vi "Client Init Test.vi"() -> (0 "no error":errorcluster, 1 "tags found":bool, 2 "expected execution settings":bool)   [LabVIEW 2013, in "OPC UA Client Tests.lvlib"]
doc: "Tests Init override for server configuration"
uses:
  OPC UA Client Tests.lvlib
  <vilib>/NI/Tag Bus/dictionary/data dictionary.lvclass
  module/configuration/OPC UA Client configuration.lvclass
  <vilib>/opcua/NI OPC UA Server.lvlib
  module/execution/OPC UA Client runtime.lvclass
  <vilib>/OPCUA/server/subVI/supported security policies.ctl
  <vilib>/NI/Tag Bus Module Framework/channel/TBM channel.lvclass
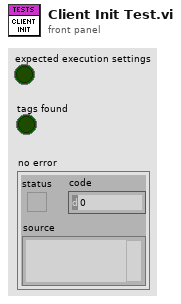
[diagram p1: front panel]
types:
  T1 = typedef "supported security policies.ctl" = cluster{"None":bool, "Sign with Basic128Rsa125":bool, "Sign and Encrypt with Basic128Rsa125":bool, "Sign with Basic256":bool, "Sign and Encrypt with Basic256":bool}
  T2 = cluster{"Client?":bool, "Server Certificates":cluster{"Relative Path?":bool, "Certificate Paths":path[], "Certificate Names":string[]}, "Client Certificates":cluster{"Relative Path?":bool, "Certificate Paths":path[], "Certificate Names":string[]}, "Client Configuration":cluster{"Server Endpoint URL":string, "Security Policy":cluster{"Message Mode":enum16{"None", "Sign", "Sign and Encrypt"}, "Security":enum16{"Basic256", "Basic128Rsa15"}}, "Username/Password":cluster{"Username":string, "Password":string}}, "Server Configuration":cluster{"Server Name":string, "TCP port (49580)":string, "Supported Security Policies":T1}}
  T3 = cluster{"Server Certificates":cluster{"Relative Path?":bool, "Certificate Paths":path[], "Certificate Names":string[]}, "Client Certificates":cluster{"Relative Path?":bool, "Certificate Paths":path[], "Certificate Names":string[]}, "Client Configuration":cluster{"Server Endpoint URL":string, "Security Policy":cluster{"Message Mode":enum16{"None", "Sign", "Sign and Encrypt"}, "Security":enum16{"Basic256", "Basic128Rsa15"}}, "Username/Password":cluster{"Username":string, "Password":string}}}
  T4 = typedef "OPC UA configuration.lvclass/Line.ctl" = cluster{"channel":refnum<class "TBM channel.lvclass">, "Node Path":string, "OPC UA Data Type":T5}
  T5 = typedef "OPC UA configuration.lvclass/OPC UA Data Type.ctl" = u16
  T6 = typedef "TBM channel.lvclass/data tables.ctl" = cluster{"input data":T7, "processing parameter":T7, "processing result":T7, "output data":T7}
  T7 = typedef "tag bus.lvlib/dictionary table pair.ctl" = cluster{"data dictionary":refnum<class "data dictionary.lvclass">, "data table":T8}
  T8 = typedef "tag bus.lvlib/data table.lvlib/data table.ctl" = cluster{"Double":dbl[], "Single":sgl[], "I64":i64[], "I32":i32[], "I16":i16[], "I8":i8[], "U64":u64[], "U32":u32[], "U16":u16[], "U8":u8[], "Boolean":bool[], "String":string[], "Array of Double":cluster{"DBL Array":dbl[]}[], "Array of Single":cluster{"SGL Array":sgl[]}[], "Array of I64":cluster{"I64 Array":i64[]}[], "Array of I32":cluster{"I32 Array":i32[]}[], "Array of I16":cluster{"I16 Array":i16[]}[], "Array of I8":cluster{"I8 Array":i8[]}[], "Array of U64":cluster{"U64 Array":u64[]}[], "Array of U32":cluster{"U32 Array":u32[]}[], "Array of U16":cluster{"U16 Array":u16[]}[], "Array of U8":cluster{"U8 Array":u8[]}[], "Array of Boolean":cluster{"Boolean Array":bool[]}[], "Array of String":cluster{"String Array":string[]}[]}
  T9 = typedef "TBM module execution interface.lvclass/execution settings.ctl" = cluster{"reads inputs":bool, "processes data":bool, "writes outputs":bool}
  T10 = typedef "tag bus.lvlib/tag descriptor.lvclass/Data Type.ctl" = enum16{"Double", "Single", "I64", "I32", "I16", "I8", "U64", "U32", "U16", "U8", "Boolean", "String", "Array of Double", "Array of Single", "Array of I64", "Array of I32", "Array of I16", "Array of I8", "Array of U64", "Array of U32", "Array of U16", "Array of U8", "Array of Boolean", "Array of String"}
  T11 = typedef "TBM channel.lvclass/channel classification.ctl" = enum16{"input data", "output data", "processing parameter", "processing result"}
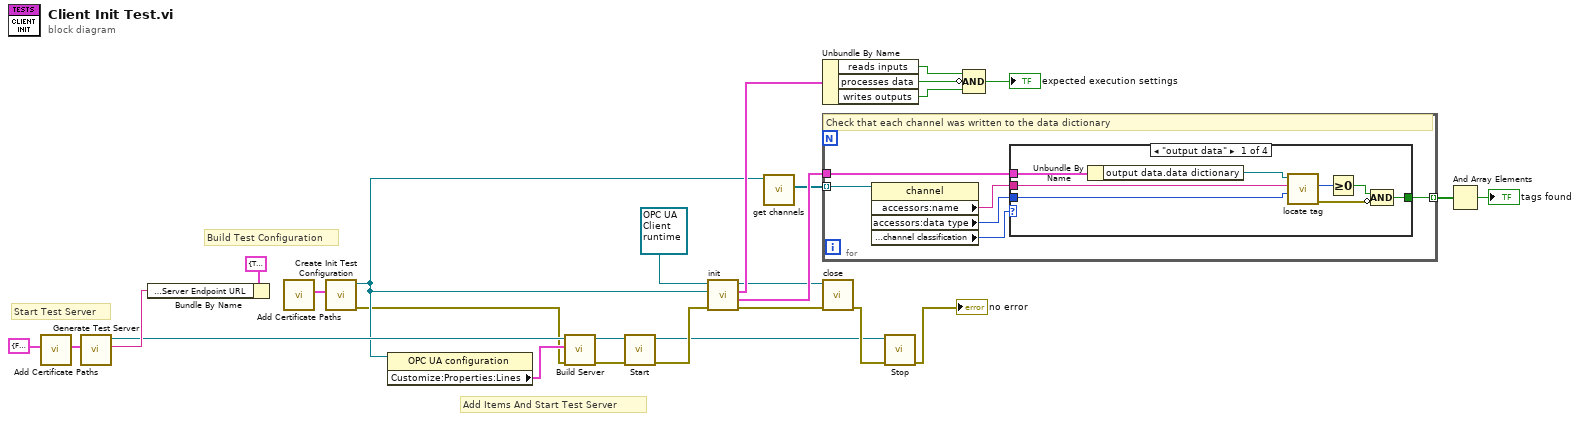
[diagram p0: block diagram]
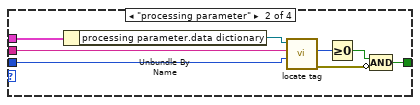
[diagram p2: hidden frame]
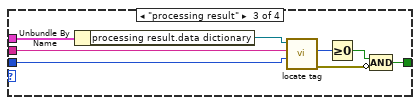
[diagram p3: hidden frame]
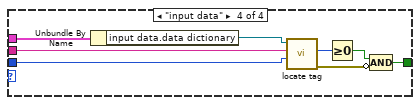
[diagram p4: hidden frame]
diagram:
  # "Add Items And Start Test Server"
  # "Start Test Server"
  # "Build Test Configuration"
  n1 = call "Add Certificate Paths.vi"("Connection Configuration In"=T2 {"Client?"=FALSE, "Server Certificates"={"Relative Path?"=FALSE, "Certificate Paths"=[path "C:/Users/Administrator/Desktop/OPC-UA-master/OPC-UA-master/Source/testing/Custom OPC UA Tests/Certificates/My Server.der"], "Certificate Names"=[]}, "Client Certificates"={"Relative Path?"=FALSE, "Certificate Paths"=[path "C:/Users/Administrator/Desktop/OPC-UA-master/OPC-UA-master/Source/testing/Custom OPC UA Tests/Certificates/DCAF Client Test Certificate.der"], "Certificate Names"=[]}, "Client Configuration"={"Server Endpoint URL"="", "Security Policy"={"Message Mode"=enum."None", "Security"=enum."Basic256"}, "Username/Password"={"Username"="", "Password"=""}}, "Server Configuration"={"Server Name"="Test", "TCP port (49580)"="49580", "Supported Security Policies"={"None"=TRUE, "Sign with Basic128Rsa125"=FALSE, "Sign and Encrypt with Basic128Rsa125"=FALSE, "Sign with Basic256"=FALSE, "Sign and Encrypt with Basic256"=FALSE}}} ("Connection Configuration")) -> ("Connection Configuration Out"=w14:T3)  [unwired: 10 in]
  n2 = call "Generate Test Server.vi"("Connection Configuration"=w14) -> ("OPC UA server refnum out"=w12:refnum<k21>, "server endpoint URL"=w13:string)  [unwired: 7 in, 1 out]
  n3 = Bundle By Name(cluster=T2 {"Client?"=TRUE, "Server Certificates"={"Relative Path?"=FALSE, "Certificate Paths"=[path "C:/Users/Administrator/Desktop/OPC-UA-master/OPC-UA-master/Source/testing/Custom OPC UA Tests/Certificates/My Server.der"], "Certificate Names"=[]}, "Client Certificates"={"Relative Path?"=FALSE, "Certificate Paths"=[path "C:/Users/Administrator/Desktop/OPC-UA-master/OPC-UA-master/Source/testing/Custom OPC UA Tests/Certificates/DCAF Client Test Certificate.der"], "Certificate Names"=[]}, "Client Configuration"={"Server Endpoint URL"="", "Security Policy"={"Message Mode"=enum."None", "Security"=enum."Basic256"}, "Username/Password"={"Username"="", "Password"=""}}, "Server Configuration"={"Server Name"="Test", "TCP port (49580)"="49580", "Supported Security Policies"={"None"=TRUE, "Sign with Basic128Rsa125"=FALSE, "Sign and Encrypt with Basic128Rsa125"=FALSE, "Sign with Basic256"=FALSE, "Sign and Encrypt with Basic256"=FALSE}}} ("Connection Configuration"), "Client Configuration.Server Endpoint URL"=w13) -> ()  [unwired: 1 out]
  n4 = call "Add Certificate Paths.vi"() -> ("Connection Configuration Out"=w1:T3)  [unwired: 11 in]
  n5 = call "Create Init Test Configuration.vi"("Connection Configuration"=w1) -> ("error out"=w9:errorcluster, "module"=w11:refnum<class "OPC UA Client configuration.lvclass">)  [unwired: 9 in]
  n6 = property class="OPC UA configuration"(reference=w11) -> ("Customize:Properties:Lines"=w10:T4[])  [unwired: 1 in, 2 out]
  n7 = call "Build Server.vi"("Error In"=w9, "Lines"=w10, "OPC UA server refnum in"=w12) -> ("Error Out"=w8:errorcluster, "OPC UA server refnum out"=w4:refnum<k21>)  [unwired: 7 in]
  n8 = call <vilib>:"Start.vi"("error in (no error)"=w8, "OPC UA server refnum in"=w4) -> ("error out"=w5:errorcluster, "OPC UA server refnum out"=w3:refnum<k21>)  [unwired: 8 in]
  n9 = call-dynamic "init.vi"("error in"=w5, "TBM module configuration in"=w11, "OPC UA runtime in"=refnum<class "OPC UA Client runtime.lvclass"> refnum ("OPC UA runtime")) -> ("error out"=w19:errorcluster, "data allocations"=w27:T6, "execution settings"=w26:T9, "OPC UA runtime out"=w16:refnum<class "OPC UA Client runtime.lvclass">)  [unwired: 5 in]
  n10 = call-dynamic "get channels.vi"("OPC UA configuration in"=w11) -> ("channels"=w18:refnum<class "TBM channel.lvclass">[])  [unwired: 9 in, 1 out]
  n11 = Unbundle By Name(w26) -> ("reads inputs"=w25:bool, "processes data"=w23:bool, "writes outputs"=w24:bool)
  n12 = for {
    tunnel: w27 -> [w33]
    tunnel: w18 -> [w32] mode=indexing
    tunnel: [w31] -> w21 mode=indexing
    # "Check that each channel was written to the data dictionary"
    n13 = property class="channel"(reference=w32) -> ("accessors:name"=w28:string, "accessors:data type"=w29:T10, "data access:channel classification"=w30:T11)  [unwired: 1 in, 2 out]
    n14 = case shown="\"output data\"" w30 {
      tunnel: w33 -> [w41 w49 w57 w65]
      tunnel: w29 -> [w39 w47 w55 w63]
      tunnel: w28 -> [w38 w46 w54 w62]
      tunnel: [w34 w42 w50 w58] -> w31
      frame "output data" {
        n15 = Unbundle By Name(w41) -> ("output data.data dictionary"=w40:refnum<class "data dictionary.lvclass">)
        n16 = call <vilib>:"locate tag.vi"("data type"=w39, "name"=w38, "data dictionary in"=w40) -> ("error out"=w35:errorcluster, "index"=w37:i32)  [unwired: 6 in, 1 out]
        n17 = Greater Or Equal To 0?(x=w37) -> (x >= 0?=w36:bool)
        n18 = Compound Arithmetic op=AND(w36, invert w35) -> (w34:bool)
      }
      frame "processing parameter" {
        n19 = Unbundle By Name(w49) -> ("processing parameter.data dictionary"=w48:refnum<class "data dictionary.lvclass">)
        n20 = call <vilib>:"locate tag.vi"("data type"=w47, "name"=w46, "data dictionary in"=w48) -> ("error out"=w43:errorcluster, "index"=w45:i32)  [unwired: 6 in, 1 out]
        n21 = Greater Or Equal To 0?(x=w45) -> (x >= 0?=w44:bool)
        n22 = Compound Arithmetic op=AND(w44, invert w43) -> (w42:bool)
      }
      frame "processing result" {
        n23 = Unbundle By Name(w57) -> ("processing result.data dictionary"=w56:refnum<class "data dictionary.lvclass">)
        n24 = call <vilib>:"locate tag.vi"("data type"=w55, "name"=w54, "data dictionary in"=w56) -> ("error out"=w51:errorcluster, "index"=w53:i32)  [unwired: 6 in, 1 out]
        n25 = Greater Or Equal To 0?(x=w53) -> (x >= 0?=w52:bool)
        n26 = Compound Arithmetic op=AND(w52, invert w51) -> (w50:bool)
      }
      frame "input data" {
        n27 = Unbundle By Name(w65) -> ("input data.data dictionary"=w64:refnum<class "data dictionary.lvclass">)
        n28 = call <vilib>:"locate tag.vi"("data type"=w63, "name"=w62, "data dictionary in"=w64) -> ("error out"=w59:errorcluster, "index"=w61:i32)  [unwired: 6 in, 1 out]
        n29 = Greater Or Equal To 0?(x=w61) -> (x >= 0?=w60:bool)
        n30 = Compound Arithmetic op=AND(w60, invert w59) -> (w58:bool)
      }
    }
  }
  n31 = call-dynamic "close.vi"("error in"=w19, "OPC UA runtime in"=w16) -> ("error out"=w7:errorcluster)  [unwired: 9 in]
  n32 = call <vilib>:"Stop.vi"("error in (no error)"=w7, "OPC UA server refnum in"=w3) -> ("error out"=→"no error":errorcluster)  [unwired: 8 in, 1 out]
  n33 = Compound Arithmetic op=AND(w25, invert w23, w24) -> (→"expected execution settings":bool)
  n34 = And Array Elements(Boolean array=w21) -> (logical AND=→"tags found":bool)
